vi "Cmd Create Parameters.vi"(4 "error in (no error)":errorcluster, 5 "parameters":T1[](array[typedef]), 6 "ADODB.Parameters":refnum<k7>, 7 "ADODB._Command":refnum<k7>) -> (0 "error out":errorcluster, 2 "ADODB.Parameters out":refnum<k7>, 3 "ADODB._Command out":refnum<k7>)   [LabVIEW 2012, in "NI_Database_API_64.lvlib"]
doc: "Creates the parameters defined by the information contained in the array for the database connection defined by the command and parameter refnums."
uses:
  NI_Database_API_64.lvlib
  Auxilliary.llb/DB Tools Parameter Info.ctl
  Auxilliary.llb/DB Tools DataTypes.ctl
  Auxilliary.llb/DB Tools Parameter Dir.ctl
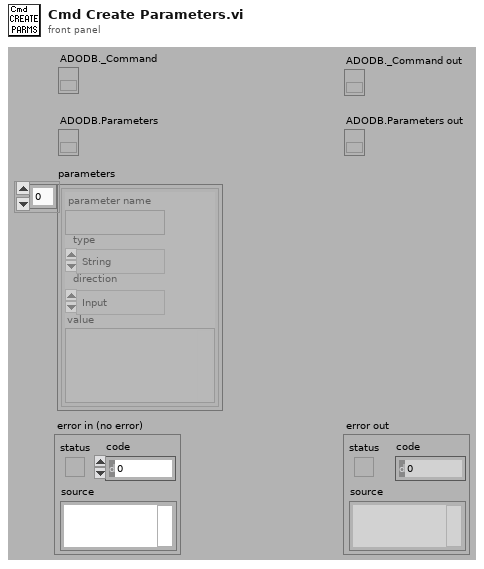
[diagram p1: front panel]
types:
  T1 = typedef "NI_Database_API_64.lvlib/DB Tools Parameter Info.ctl" = cluster{"parameter name":string, "type":T2, "direction":T3, "value":variant}
  T2 = typedef "NI_Database_API_64.lvlib/DB Tools DataTypes.ctl" = enum16{"String", "Long (I32)", "Single (SGL)", "Double (DBL)", "Date/Time", "Binary"}
  T3 = typedef "NI_Database_API_64.lvlib/DB Tools Parameter Dir.ctl" = enum32{"Input", "Output", "Input/Output", "Return Value"}
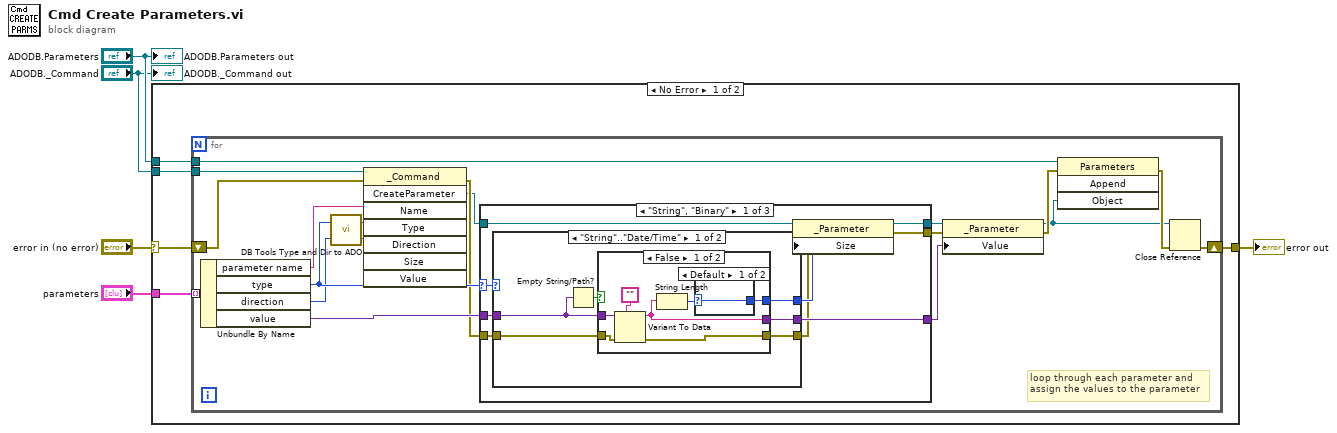
[diagram p0: block diagram]
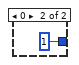
[diagram p2: hidden frame]
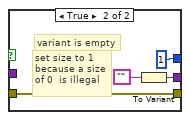
[diagram p3: hidden frame]
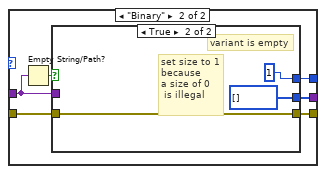
[diagram p4: hidden frame]
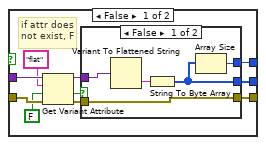
[diagram p5: hidden frame]
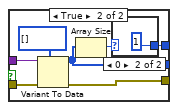
[diagram p6: hidden frame]
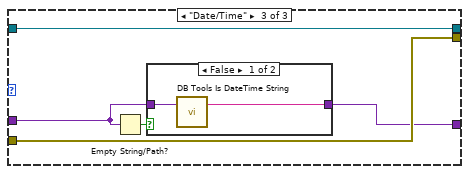
[diagram p9: hidden frame]
diagram:
  n1 = case shown="No Error" "error in (no error)" {
    selector: "error in (no error)" -> [w6 w102]
    tunnel: "ADODB.Parameters" -> [w10 _]
    tunnel: "ADODB._Command" -> [w9 _]
    tunnel: [w8 w102] -> w5
    tunnel: "parameters" -> [w7 _]
    frame No Error {
      n2 = for {
        tunnel: w9 -> [w17]
        tunnel: w10 -> [w29]
        shift-right: [w27] -> w8
        shift-left: w6 -> [w16]
        tunnel: w7 -> [w26] mode=indexing
        # "loop through each parameter and\nassign the values to the parameter"
        n3 = Unbundle By Name(w26) -> ("parameter name"=w15:string, "type"=w22:T2, "direction"=w21:T3, "value"=w25:variant)
        n4 = call "DB Tools Type and Dir to ADO.vi"("direction"=w21, "data type"=w22) -> ("ADO direction"=w13:u16, "ADO type"=w14:u16)
        n5 = invoke class="_Command" method="CreateParameter"(reference=w17, error in=w16, "Name"=w15, "Type"=w14, "Direction"=w13) -> (error out=w12:errorcluster, "CreateParameter"=w11:refnum<k7>)  [unwired: 3 in, 6 out]
        n6 = case shown="\"String\", \"Binary\"" w22 {
          selector: w22 -> [w34 _ _]
          tunnel: w25 -> [w33 w91 w94]
          tunnel: [w38 w93 w98] -> w24
          tunnel: [w37 w92 w97] -> w23
          tunnel: w11 -> [w36 w93 w98]
          tunnel: w12 -> [w32 w92 w97]
          tunnel: [w31 w91 w96] -> w18
          frame "String", "Binary" {
            n7 = case shown="\"String\"..\"Date/Time\"" w34 {
              tunnel: [w43 w62] -> w35
              tunnel: w33 -> [w42 w59]
              tunnel: w32 -> [w41 w58]
              tunnel: [w40 w61] -> w30
              tunnel: [w39 w60] -> w31
              frame "String".."Date/Time" {
                n8 = Empty String/Path?(string/path=w42) -> (empty?=w44:bool)
                n9 = case shown="False" w44 {
                  tunnel: [w50 1] -> w43
                  tunnel: w42 -> [w49 _]
                  tunnel: w41 -> [w48 w56]
                  tunnel: [w47 w56] -> w40
                  tunnel: [w45 w54] -> w39
                  frame False {
                    n10 = Variant To Data(error in=w48, type="", Variant=w49) -> (data=w45:string, error out=w47:errorcluster)
                    n11 = String Length(string=w45) -> (length=w51:i32)
                    n12 = case shown="Default" w51 {
                      selector: w51 -> [w52 _]
                      tunnel: [w52 1] -> w50
                      frame Default {
                      }
                      frame 0 {
                      }
                    }
                  }
                  frame True {
                    # "set size to 1 \nbecause a size \nof 0  is illegal"
                    # "variant is empty"
                    n13 = To Variant(anything="") -> (Variant=w54:variant)
                  }
                }
              }
              frame "Binary" {
                n14 = Empty String/Path?(string/path=w59) -> (empty?=w63:bool)
                n15 = case shown="True" w63 {
                  tunnel: [w72 1] -> w62
                  tunnel: w58 -> [w69 w89]
                  tunnel: [w73 w89] -> w61
                  tunnel: [w71 u8[] [] ("Array Constant")] -> w60
                  tunnel: w59 -> [w70 _]
                  frame False {
                    # "if attr does\nnot exist, F"
                    n16 = Get Variant Attribute(Variant=w70, name="flat", default value (empty Variant)=FALSE, error in=w69) -> (duplicate Variant=w64:variant, value=w66:bool, error out=w65:errorcluster)  [unwired: 1 out]
                    n17 = case shown="False" w66 {
                      tunnel: [w74 w85] -> w73
                      tunnel: [w75 w80] -> w72
                      tunnel: [w76 w83] -> w71
                      tunnel: w64 -> [w78 w82]
                      tunnel: w65 -> [w74 w81]
                      frame False {
                        n18 = Variant To Flattened String(Variant=w78) -> (data string=w77:string)  [unwired: 1 out]
                        n19 = String To Byte Array(string=w77) -> (unsigned byte array=w76:u8[])
                        n20 = Array Size(array=w76) -> (size(s)=w75:i32)
                      }
                      frame True {
                        n21 = Variant To Data(error in=w81, type=u8[] [] ("Array Constant"), Variant=w82) -> (data=w83:u8[], error out=w85:errorcluster)
                        n22 = Array Size(array=w83) -> (size(s)=w79:i32)
                        n23 = case shown="0" w79 {
                          selector: w79 -> [w86 _]
                          tunnel: [w86 1] -> w80
                          frame Default {
                          }
                          frame 0 {
                          }
                        }
                      }
                    }
                  }
                  frame True {
                    # "set size to 1 \nbecause\na size of 0\n is illegal"
                    # "variant is empty"
                  }
                }
              }
            }
            n24 = property class="_Parameter"(reference=w36, error in=w30, "Size"=w35) -> (reference out=w38:refnum<k7>, error out=w37:errorcluster)
          }
          frame "Long (I32)".."Double (DBL)" {
          }
          frame "Date/Time" {
            n25 = Empty String/Path?(string/path=w94) -> (empty?=w95:bool)
            n26 = case shown="False" w95 {
              tunnel: [w99 w101] -> w96
              tunnel: w94 -> [w100 w101]
              frame False {
                n27 = call "DB Tools Is DateTime String.vi"("string or date/time"=w100) -> ("data"=w99:string)  [unwired: 1 in, 1 out]
              }
              frame True {
              }
            }
          }
        }
        n28 = property class="_Parameter"(reference=w24, error in=w23, "Value"=w18) -> (reference out=w19:refnum<k7>, error out=w20:errorcluster)
        n29 = invoke class="Parameters" method="Append"(reference=w29, error in=w20, "Object"=w19) -> (error out=w28:errorcluster)  [unwired: 1 in, 3 out]
        n30 = Close Reference(reference=w19, error in (no error)=w28) -> (error out=w27:errorcluster)
      }
    }
    frame Error {
    }
  }
  "error out" <- w5
  "ADODB._Command out" <- "ADODB._Command"
  "ADODB.Parameters out" <- "ADODB.Parameters"
